vi "PicoScope6000GetValuesOverlapped.vi"(5 "Segment Range":T1 {"toSegmentIndex" format="%.4p"; "fromSegmentIndex" format="%.4p"}, 7 "Buffer and Transfer Settings":T2 {"Down-Sample Mode" items=["RAW none", "None", "Aggregate", "Decimate", "Average"]; "Down Sample Ratio" step=1; "Samples" format="%_6p"}, 8 "error in (no error)":errorcluster, 11 "handle in":i16) -> (0 "error out":errorcluster, 3 "handle out":i16, 4 "Pointer to Overflow":u64[](array[numeric]) format="%010b", 6 "noOfSamples":u64)   [LabVIEW 2009]
doc: "Calls ps5000aGetValuesOverlapped"
uses:
  ps6000.dll
  shared/Segment Range.ctl
  shared/Buffer and Transfer Settings.ctl
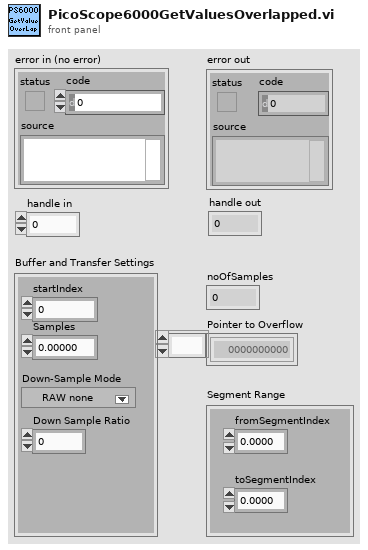
[diagram p1: front panel]
types:
  T1 = typedef "Segment Range.ctl" = cluster{"fromSegmentIndex":u64, "toSegmentIndex":u64}
  T2 = typedef "Buffer and Transfer Settings.ctl" = cluster{"startIndex":u64, "Samples":u64, "Down Sample Ratio":u64, "Down-Sample Mode":u32}
  T3 = cluster{"status":bool, "code":u32, "source":string}
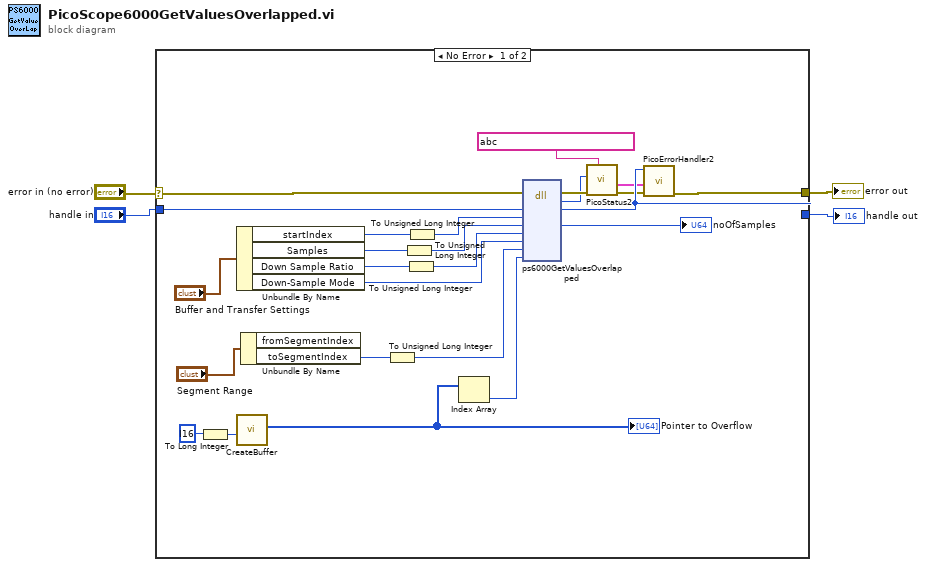
[diagram p0: block diagram]
diagram:
  n1 = case shown="No Error" "error in (no error)" {
    selector: "error in (no error)" -> [w27 w30]
    tunnel: "handle in" -> [w26 w31]
    tunnel: [w24 w31] -> w4
    tunnel: [w25 w30] -> w3
    frame #0 {
      n2 = To Long Integer(number=i16 ? ("overflow")) -> (32bit integer=w8:i32)
      n3 = Unbundle By Name("Buffer and Transfer Settings") -> ("startIndex"=w16:u64, "Samples"=w14:u64, "Down Sample Ratio"=w12:u64, "Down-Sample Mode"=w29:u32)
      n4 = call "CreateBuffer.vi"("Buffer size"=w8) -> ("Pointer and BufferSize"=w5:u64[])  [unwired: 9 in, 1 out]
      "Pointer to Overflow" <- w5
      n5 = Unbundle By Name("Segment Range") -> ("toSegmentIndex"=w10:u64)  [unwired: 1 out]
      n6 = To Unsigned Long Integer(number=w10) -> (unsigned 32bit integer=w9:u32)
      n7 = To Unsigned Long Integer(number=w14) -> (unsigned 32bit integer=w13:u32)
      n8 = To Unsigned Long Integer(number=w12) -> (unsigned 32bit integer=w11:u32)
      n9 = To Unsigned Long Integer(number=w16) -> (unsigned 32bit integer=w15:u32)
      n10 = Index Array(array=w5) -> (element=w6:u64)  [unwired: 1 in]
      n11 = dll-call lib="ps6000.dll" fn="ps6000GetValuesOverlapped" ("ps3000.dll:_ps3000_open_unit@0")(error in=w27, "handle"=w26, "startIndex"=w15, "noOfSamples"=w13, "downSampleRatio"=w11, "downSampleRatioMode"=w29, "segmentIndex"=w9, "overflow"=w6) -> (error out=w20:errorcluster, "PICO_STATUS"=w17:u32, "handle"=w24:i16, "noOfSamples"=→"noOfSamples":u32)  [unwired: 7 in, 1 out]
      n12 = call "PicoStatus2.vi"("PICO source"=string ? ("source"), "Error in"=w20, "PICO STATUS"=w17) -> ("error out"=w21:errorcluster, "PICO_STATUS out"=w18:T3)  [unwired: 5 in]
      n13 = call "PicoErrorHandler2.vi"("error in (no error)"=w21, "PICO_STATUS in"=w18, "handle In"=w24) -> ("error out"=w25:errorcluster)  [unwired: 8 in]
    }
    frame #1 {
    }
  }
  "error out" <- w3
  "handle out" <- w4
